vi "RefToString.vi"(6 "StrRef":refnum<vi>) -> (1 "String":string, 2 "StrRefOut":refnum<vi>)   [LabVIEW 2013]
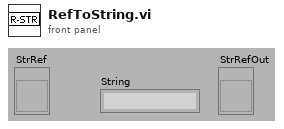
[diagram p1: front panel]
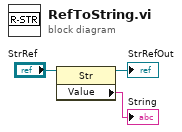
[diagram p0: block diagram]
diagram:
  n1 = property class="Str"(reference="StrRef") -> (reference out=→"StrRefOut":refnum<vi>, "Value"=→"String":string)  [unwired: 1 in, 1 out]
